vi "SFP Get DAQmx Devices Status.vi"(0 "device info":T1 {"Device Info"."Serial Number" format="%x"}, 5 "update interval":dbl format="%#_13g", 9 "status info in":variant, 11 "error in":errorcluster) -> (4 "device info":T1 {"Device Info"."Serial Number" format="%x"}, 10 "status info out":variant, 15 "error out":errorcluster)   [LabVIEW 2017]
uses:
  <vilib>/addons/Sound and Vibration/svt_DAQmx/subVIs/SFP DAQmx Device Info.ctl
  <resource>/objmgr/daqmx.rc
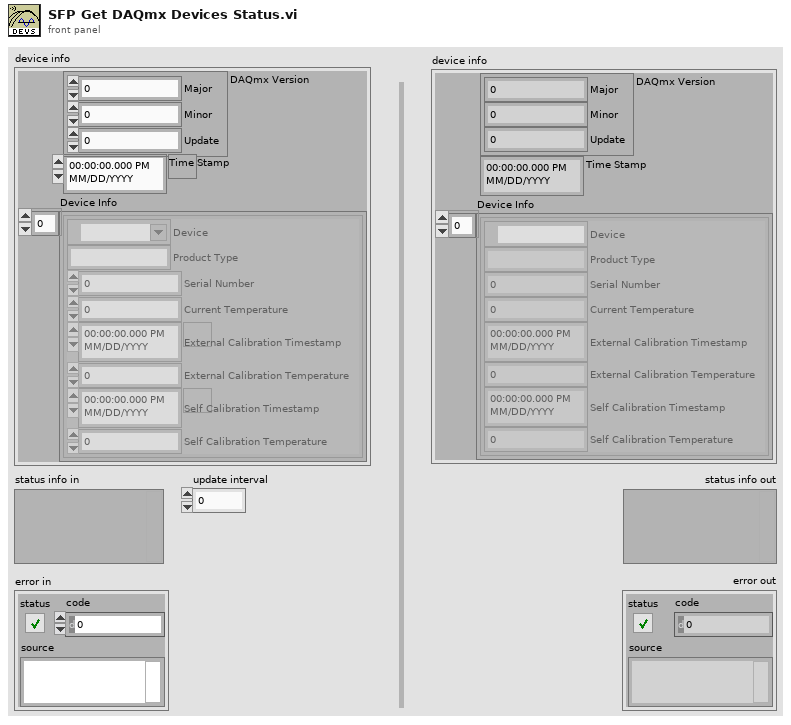
[diagram p1: front panel]
types:
  T1 = typedef "SFP DAQmx Device Info.ctl" = cluster{"DAQmx Version":cluster{"Major":u32, "Minor":u32, "Update":u32}, "Time Stamp":timestamp, "Device Info":cluster{"Device":tag, "Product Type":string, "Serial Number":u32, "Current Temperature":dbl, "External Calibration Timestamp":timestamp, "External Calibration Temperature":dbl, "Self Calibration Timestamp":timestamp, "Self Calibration Temperature":dbl}[]}
  T2 = cluster{"Device":tag, "Product Type":string, "Serial Number":u32, "Current Temperature":dbl, "External Calibration Timestamp":timestamp, "External Calibration Temperature":dbl, "Self Calibration Timestamp":timestamp, "Self Calibration Temperature":dbl}[]
  T3 = cluster{"Device":tag, "Product Type":string, "Serial Number":u32, "Current Temperature":dbl, "External Calibration Timestamp":timestamp, "External Calibration Temperature":dbl, "Self Calibration Timestamp":timestamp, "Self Calibration Temperature":dbl}
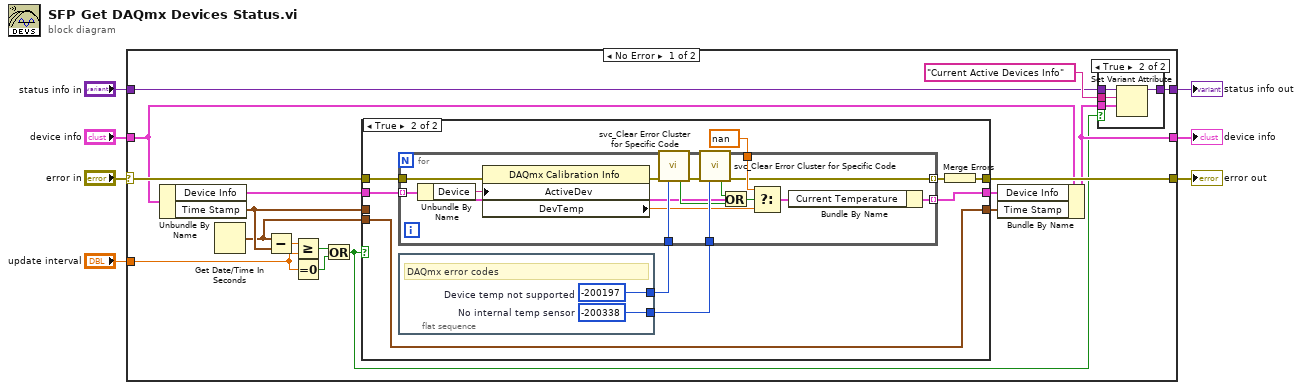
[diagram p0: block diagram]
diagram:
  n1 = case shown="No Error" "error in" {
    selector: "error in" -> [w19 w60]
    tunnel: "device info" -> [w18 w61]
    tunnel: [w12 w61] -> w6
    tunnel: [w23 w59] -> w5
    tunnel: [w21 w60] -> w4
    tunnel: "status info in" -> [w22 w59]
    tunnel: "update interval" -> [w10 _]
    frame No Error {
      n2 = Unbundle By Name(w18) -> ("Device Info"=w20:T2, "Time Stamp"=w14:timestamp)
      n3 = Get Date/Time In Seconds() -> (seconds since 1Jan1904=w13:timestamp)
      n4 = Subtract(x=w13, y=w14) -> (x-y=w16:dbl)
      n5 = Greater Or Equal?(x=w16, y=w10) -> (x >= y?=w9:bool)
      n6 = Equal To 0?(x=w10) -> (x = 0?=w11:bool)
      n7 = Or(x=w9, y=w11) -> (x .or. y?=w8:bool)
      n8 = case shown="True" w8 {
        tunnel: [w32 w37] -> w21
        tunnel: w20 -> [w31 w36]
        tunnel: w19 -> [w32 w35]
        tunnel: [w31 w34] -> w17
        tunnel: [w30 w33] -> w15
        tunnel: w13 -> [_ w33]
        tunnel: w14 -> [w30 _]
        frame False {
        }
        frame True {
          n9 = for {
            tunnel: w36 -> [w46] mode=indexing
            tunnel: w35 -> [w58]
            tunnel: w41 -> [w56]
            tunnel: w40 -> [w54]
            tunnel: nan ("t") -> [w49]
            tunnel: [w48] -> w38 mode=indexing
            tunnel: [w44] -> w34 mode=indexing
            n10 = Unbundle By Name(w46) -> ("Device"=w47:tag)
            n11 = property class="DAQmx Calibration Info"(error in=w58, "ActiveDev"=w47) -> (error out=w57:errorcluster, "DevTemp"=w50:dbl)  [unwired: 1 in, 1 out]
            n12 = call <vilib>:"svc_Clear Error Cluster for Specific Code.vi"("error in (no error)"=w57, "code"=w56) -> ("error cleared"=w52:bool, "error out"=w55:errorcluster)  [unwired: 12 in]
            n13 = call <vilib>:"svc_Clear Error Cluster for Specific Code.vi"("error in (no error)"=w55, "code"=w54) -> ("error cleared"=w53:bool, "error out"=w48:errorcluster)  [unwired: 12 in]
            n14 = Or(x=w53, y=w52) -> (x .or. y?=w51:bool)
            n15 = Select(t=w49, s=w51, f=w50) -> (s? t:f=w45:dbl)
            n16 = Bundle By Name(cluster=w46, "Current Temperature"=w45) -> (w44:T3)
          }
          n17 = flat-sequence {
            tunnel: [w43] -> w41
            tunnel: [w42] -> w40
            frame #0 {
              w42 = -200338  # No internal temp sensor
              w43 = -200197  # Device temp not supported
              # "DAQmx error codes"
            }
          }
          n18 = Merge Errors(w38) -> (w37:errorcluster)
        }
      }
      n19 = Bundle By Name(cluster=w18, "Device Info"=w17, "Time Stamp"=w15) -> (w12:T1)
      n20 = case shown="True" w8 {
        tunnel: "Current Active Devices Info" ("name") -> [_ w29]
        tunnel: [w25 w28] -> w23
        tunnel: w22 -> [w25 w27]
        tunnel: w12 -> [_ w26]
        frame False {
        }
        frame True {
          n21 = Set Variant Attribute(Variant=w27, name=w29, value=w26) -> (Variant out=w28:variant)  [unwired: 1 in, 2 out]
        }
      }
    }
    frame Error {
    }
  }
  "status info out" <- w5
  "error out" <- w4
  "device info" <- w6
